vi "ConfigInstr.vi"(6 "InstrumentName":string, 7 "VisaRessIn":refnum<visa-resource-name>="GPIB0::12::INSTR", 8 "error in (no error)":errorcluster caption="entrée d'erreur (pas d'erreur)", 9 "FirstClassInst":bool, 10 "Function":string, 11 "EG_G5210 In":refnum<class "EG_G5210.lvclass"> caption="DNL_LabVIEW Object in") -> (0 "error out":errorcluster caption="sortie d'erreur", 3 "EG_G5210 Out":refnum<class "EG_G5210.lvclass"> caption="DNL_LabVIEW Object out")   [LabVIEW 2010, in "EG_G5210.lvclass"]
uses:
  EG_G5210.lvclass
  EG_G5210_Func.ctl
  EG_G5210.lvclass/EG_G5210.ctl
  BaseDevice/BaseDevice.lvclass
panel:
  in  "EG_G5210_Func":T1
  out "VisaRessOut":refnum<visa-resource-name>
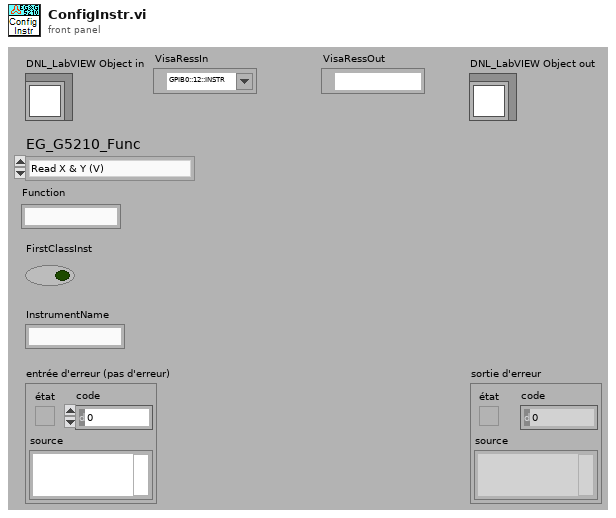
[diagram p1: front panel]
types:
  T1 = typedef "EG_G5210.lvclass/EG_G5210_Func.ctl" = enum16{"Read X & Y (V)", "Read Mag & Phase (V,°)", "Read X, Y, Mag & Phase (V,V,V,°)", "Read ADC Ch1 (V)", "Read ADC Ch2 (V)"}
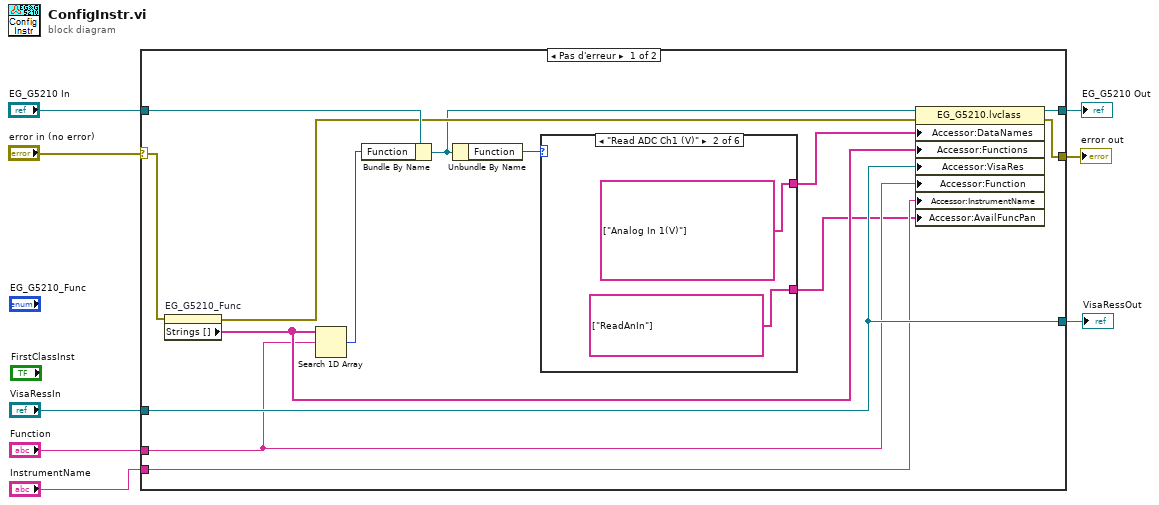
[diagram p0: block diagram]
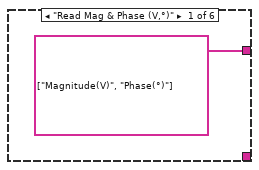
[diagram p2: hidden frame]
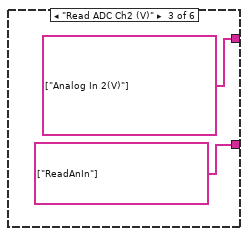
[diagram p3: hidden frame]
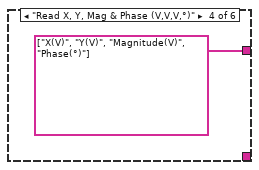
[diagram p4: hidden frame]
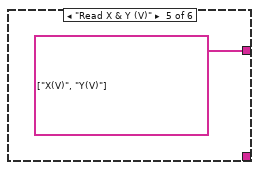
[diagram p5: hidden frame]
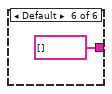
[diagram p6: hidden frame]
diagram:
  n1 = case shown="Pas d'erreur" "error in (no error)" {
    selector: "error in (no error)" -> [w19 w32]
    tunnel: [w17 w32] -> w7
    tunnel: "EG_G5210 In" -> [w21 w31]
    tunnel: [w18 w31] -> w5
    tunnel: "Function" -> [w11 _]
    tunnel: "VisaRessIn" -> [w13 _]
    tunnel: [w13 _] -> w2
    tunnel: "InstrumentName" -> [w10 _]
    frame No Error {
      n2 = property on="EG_G5210_Func" class="Énum (strict)"(error in=w19) -> (error out=w20:errorcluster, "Strings []"=w12:string[])  [unwired: 1 in, 1 out]
      n3 = Search 1D Array(1D array=w12, element=w11) -> (index of element=w22:i32)  [unwired: 1 in]
      n4 = Bundle By Name(cluster=w21, "Function"=w22) -> (w16:refnum<class "EG_G5210.lvclass">)
      n5 = Unbundle By Name(w16) -> ("Function"=w15:T1)
      n6 = case shown="\"Read ADC Ch1 (V)\"" w15 {
        tunnel: [string[] ["Magnitude(V)", "Phase(°)"] string[] ["Analog In 1(V)"] string[] ["Analog In 2(V)"] string[] ["X(V)", "Y(V)", "Magnitude(V)", "Phase(°)"] string[] ["X(V)", "Y(V)"] string[] []] -> w14
        tunnel: [_ string[] ["ReadAnIn"] string[] ["ReadAnIn"] _ _ _] -> w9
        frame "Read Mag & Phase (V,°)" {
        }
        frame "Read ADC Ch1 (V)" {
        }
        frame "Read ADC Ch2 (V)" {
        }
        frame "Read X, Y, Mag & Phase (V,V,V,°)" {
        }
        frame "Read X & Y (V)" {
        }
        frame Default {
        }
      }
      n7 = property class="EG_G5210.lvclass"(reference=w16, error in=w20, "Accessor:DataNames"=w14, "Accessor:Functions"=w12, "Accessor:VisaRes"=w13, "Accessor:Function"=w11, "Accessor:InstrumentName"=w10, "Accessor:AvailFuncPan"=w9) -> (reference out=w18:refnum<class "EG_G5210.lvclass">, error out=w17:errorcluster)
    }
    frame Error {
    }
  }
  "error out" <- w7
  "EG_G5210 Out" <- w5
  "VisaRessOut" <- w2
